vi "Suspected Pixels Tester.vi"() -> ()   [LabVIEW 2015]
uses:
  IP results.ctl
  <vilib>/Analysis/NI_AALBase.lvlib
panel:
  out "median 2":dbl=392.0 format="%0.2f"
  out "median":dbl=298.0 format="%0.2f"
  out "Array 2":u32[](array[numeric])=[138, 138, 138, 139, 139, 141, 141, 143, 143, 146, 146, 149, 149, 153, 153, 158, 158, 163, 163, 169, 169, 175, 175, 181, 181, 188, 188, 196, 196, 204, 204, 212, 212, 221, 221, 230, 230, 239, 239, 249, 249, 258, 258, 268, 268, 278, 278, 288, 288, 298, 298, 308, 308, 318, 318, 328, 328, 338, 338, 347, 347, 357, 357, 366, 366, 375, 375, 384, 384, 392, 392, 400, 400, 408, 408, 415, 415, 421, 421, 427, 427, 433, 433, 438, 438, 443, 443, 447, 447, 450, 450, 453, 453, 455, 455, 457, 457, 458, 458, 458]
  out "Array":u32[](array[numeric])=[383, 392, 401, 373, 411, 364, 420, 355, 429, 346, 438, 337, 447, 328, 456, 320, 464, 312, 472, 304, 480, 296, 488, 289, 495, 283, 501, 276, 508, 271, 513, 265, 519, 261, 523, 256, 528, 253, 531, 249, 535, 247, 537, 245, 539, 243, 541, 242, 542, 242, 542, 242, 542, 243, 541, 245, 539, 247, 537, 249, 535, 253, 531, 256, 528, 261, 523, 265, 519, 271, 513, 276, 508, 283, 501, 289, 495, 296, 488, 304, 480, 312, 472, 320, 464, 328, 456, 337, 447, 346, 438, 355, 429, 364, 420, 373, 411, 383, 392, 401]
  out "Numeric":u32=100
  out "Image Out 2":T1(plugin-control)
  in  "IP Results 2":T2={"X"=392, "Y"=298, "A"=150.0, "B"=160.0, "Grade"=0, "Frame#"=0}
  out "size(s)":i32=21776
  out "SuspPixelsIndex":u32[](array[numeric])
  out "Image Out":T1(plugin-control)
  out "Y Points":i16[](array[numeric])=[0, 10, 20, 30, 40, 49, 59, 68, 77, 86, 94, 102, 110, 117, 123, 129, 135, 140, 145, 149, 152, 155, 157, 159, 160, 160, 160, 159, 157, 155, 152, 149, 145, 140, 135, 129, 123, 117, 110, 102, 94, 86, 77, 68, 59, 49, 40, 30, 20, 10, 0, -10, -20, -30, -40, -49, -59, -68, -77, -86, -94, -102, -110, -117, -123, -129, -135, -140, -145, -149, -152, -155, -157, -159, -160, -160, -160, -159, -157, -155, -152, -149, -145, -140, -135, -129, -123, -117, -110, -102, -94, -86, -77, -68, -59, -49, -40, -30, -20, -10]
  out "X Points":i16[](array[numeric])=[150, 150, 149, 147, 145, 143, 139, 136, 131, 127, 121, 116, 109, 103, 96, 88, 80, 72, 64, 55, 46, 37, 28, 19, 9, 0, -9, -19, -28, -37, -46, -55, -64, -72, -80, -88, -96, -103, -109, -116, -121, -127, -131, -136, -139, -143, -145, -147, -149, -150, -150, -150, -149, -147, -145, -143, -139, -136, -131, -127, -121, -116, -109, -103, -96, -88, -80, -72, -64, -55, -46, -37, -28, -19, -9, 0, 9, 19, 28, 37, 46, 55, 64, 72, 80, 88, 96, 103, 109, 116, 121, 127, 131, 136, 139, 143, 145, 147, 149, 150]
  in  "tolerance":i32=20
  in  "IP Results":T2={"X"=400, "Y"=300, "A"=150.0, "B"=160.0, "Grade"=0, "Frame#"=0}
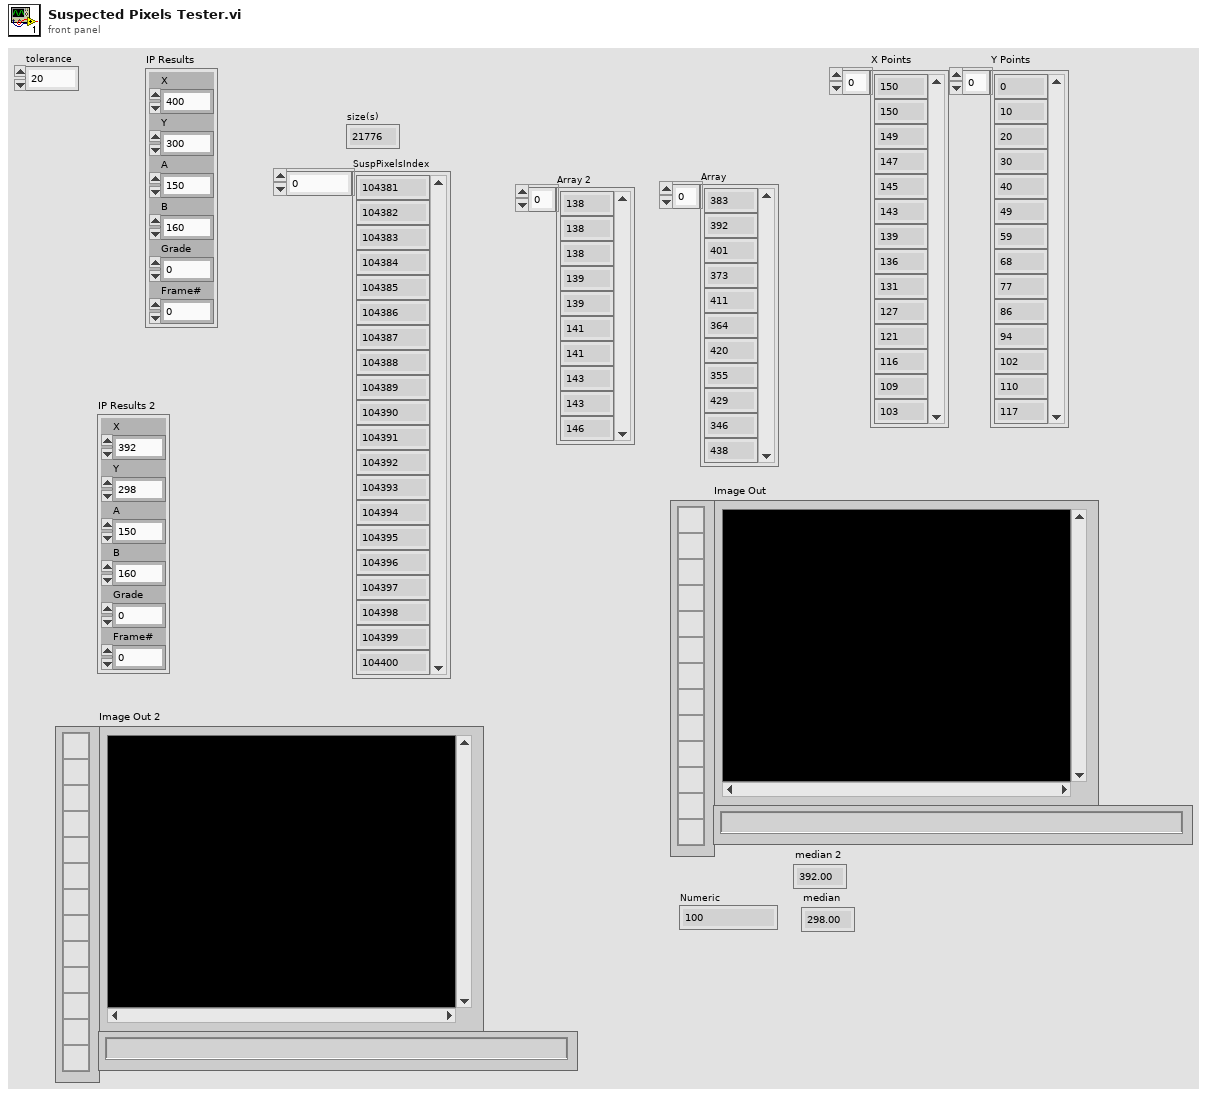
[diagram p1: front panel]
types:
  T1 = typedef "IMAQ Image.ctl" = refnum<image>
  T2 = typedef "IP results.ctl" = cluster{"X":u16, "Y":u16, "A":dbl, "B":dbl, "Grade":u16, "Frame#":u16}
  T3 = typedef "Image Type" = u32
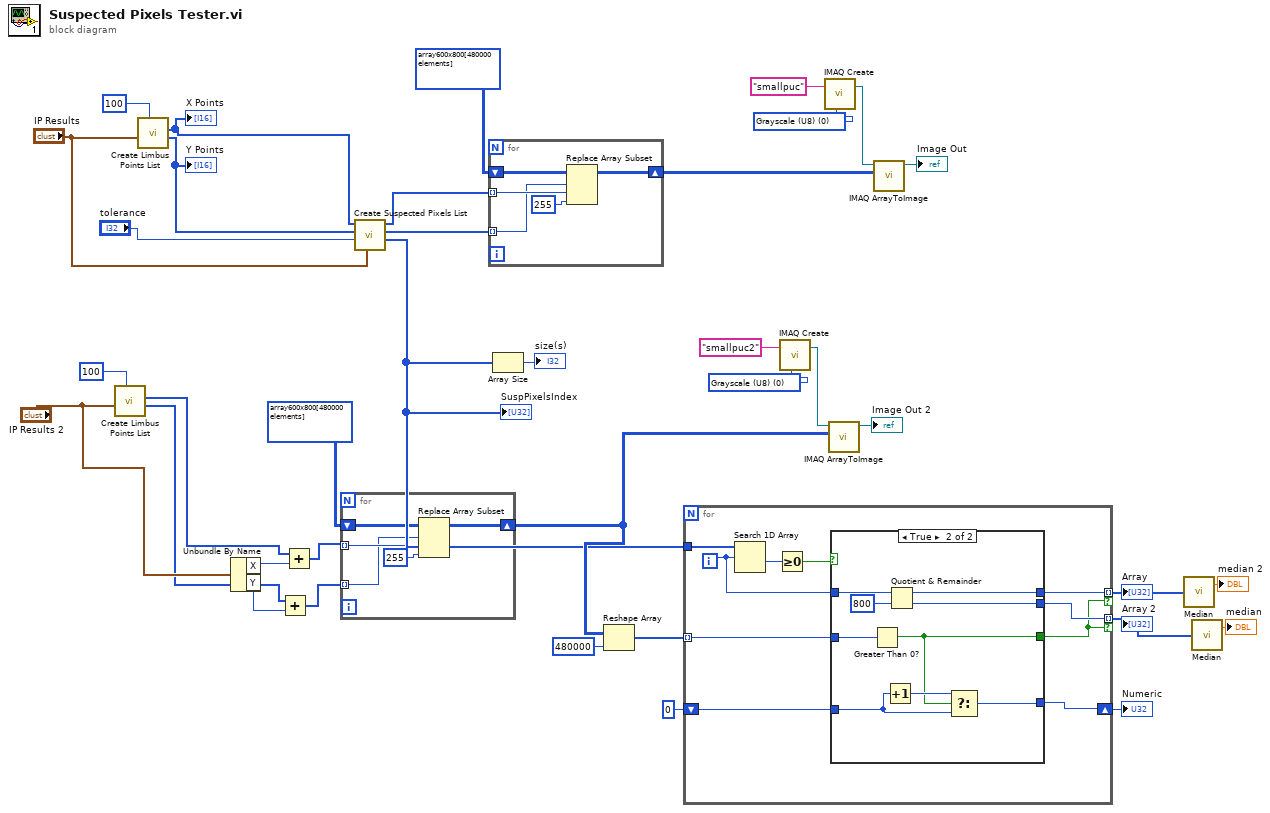
[diagram p0: block diagram]
diagram:
  w20 = T3 0 items=["Grayscale (U8)", "Grayscale (I16)", "Grayscale (SGL)", "Complex (CSG)", "RGB (U32)", "HSL (U32)", "RGB (U64)", "Grayscale (U16)"] ("Image Type")
  w31 = T3 0 items=["Grayscale (U8)", "Grayscale (I16)", "Grayscale (SGL)", "Complex (CSG)", "RGB (U32)", "HSL (U32)", "RGB (U64)", "Grayscale (U16)"] ("Image Type")
  n1 = call "Create Limbus Points List.vi"("NoOfPoints"=u16 100, "IP Results"="IP Results 2") -> ("Y Points"=w12:i16[], "X Points"=w16:i16[])  [unwired: 8 in]
  n2 = call "Create Limbus Points List.vi"("NoOfPoints"=u16 100, "IP Results"="IP Results") -> ("Y Points"=w35:i16[], "X Points"=w36:i16[])  [unwired: 8 in]
  "X Points" <- w36
  "Y Points" <- w35
  n3 = Unbundle By Name("IP Results 2") -> ("X"=w15:u16, "Y"=w13:u16)
  n4 = Add(x=w12, y=w13) -> (x+y=w11:u16[])
  n5 = Add(x=w16, y=w15) -> (x+y=w14:u16[])
  n6 = for {
    shift-right: [w41] -> w10
    shift-left: u8[][] array600x800[480000 elements] ("Image Pixels (U8)") -> [w42]
    tunnel: w14 -> [w40] mode=indexing
    tunnel: w11 -> [w39] mode=indexing
    n7 = Replace Array Subset(array=w42, new element=u8 255 ("new element/subarray"), index (row)=w39, index (col)=w40) -> (w41:u8[][])
  }
  n8 = call "Create Suspected Pixels List.vi"("IP Results"="IP Results", "tolerance"="tolerance", "Y Points"=w35, "X Points"=w36) -> ("SuspPixelsIndex"=w7:u32[], "SuspPixelsY"=w27:u32[], "SuspPixelsX"=w28:u32[])  [unwired: 5 in]
  "SuspPixelsIndex" <- w7
  n9 = for {
    shift-right: [w46] -> w26
    shift-left: u8[][] array600x800[480000 elements] ("Image Pixels (U8)") -> [w47]
    tunnel: w28 -> [w45] mode=indexing
    tunnel: w27 -> [w44] mode=indexing
    n10 = Replace Array Subset(array=w47, new element=u8 255 ("new element/subarray"), index (row)=w44, index (col)=w45) -> (w46:u8[][])
  }
  n11 = Array Size(array=w7) -> (size(s)=→"size(s)":i32)
  n12 = Reshape Array(w10, 480000 ("dimension size")) -> (w8:u8[])
  n13 = for {
    tunnel: w8 -> [w54] mode=indexing
    tunnel: w7 -> [w57]
    shift-right: [w52] -> w5
    shift-left: u32 0 -> [w53]
    tunnel: [w51] -> w1 mode=indexing if=w49
    tunnel: [w50] -> w4 mode=indexing if=w49
    i -> [w48]
    n14 = Search 1D Array(1D array=w57, element=w48) -> (index of element=w56:i32)  [unwired: 1 in]
    n15 = Greater Or Equal To 0?(x=w56) -> (x >= 0?=w55:bool)
    n16 = case shown="True" w55 {
      tunnel: w54 -> [_ w64]
      tunnel: w53 -> [w58 w67]
      tunnel: [w58 w65] -> w52
      tunnel: [_ w63] -> w51
      tunnel: [_ w62] -> w50
      tunnel: [_ w61] -> w49
      tunnel: w48 -> [_ w60]
      frame False {
      }
      frame True {
        n17 = Greater Than 0?(x=w64) -> (x > 0?=w61:bool)
        n18 = Increment(x=w67) -> (x+1=w66:u32)
        n19 = Quotient & Remainder(x=w60, y=800) -> (x-y*floor(x/y)=w63:i32, floor(x/y)=w62:i32)
        n20 = Select(t=w66, s=w61, f=w67) -> (s? t:f=w65:u32)
      }
    }
  }
  "Numeric" <- w5
  "Array" <- w1
  "Array 2" <- w4
  n21 = call "IMAQ Create"("Image Name"="smallpuc2", "Image Type"=w20) -> ("New Image"=w19:T1)  [unwired: 3 in, 1 out]
  n22 = call "IMAQ Create"("Image Name"="smallpuc", "Image Type"=w31) -> ("New Image"=w32:T1)  [unwired: 3 in, 1 out]
  n23 = call "IMAQ ArrayToImage"("Image Pixels (U8)"=w10, "Image"=w19) -> ("Image Out"=→"Image Out 2":T1)  [unwired: 8 in, 1 out]
  n24 = call "IMAQ ArrayToImage"("Image Pixels (U8)"=w26, "Image"=w32) -> ("Image Out"=→"Image Out":T1)  [unwired: 8 in, 1 out]
  n25 = call <vilib>:"Median.vi"("X"=w1) -> ("median"=→"median 2":dbl)  [unwired: 1 out]
  n26 = call <vilib>:"Median.vi"("X"=w4) -> ("median"=→"median":dbl)  [unwired: 1 out]
